vi "SetOpenDataEvents.vi"(7 "data group":string, 8 "error in (no error)":errorcluster, 9 "data event configs":T1[](array[typedef]), 10 "data events":T8[](array[typedef]), 11 "config":T7) -> (0 "error out":errorcluster, 3 "config out":T7)   [LabVIEW 2017, in "CmsDataEventCreator.lvlib"]
uses:
  <vilib>/addons/InsightCM/Devices/Shared/Cms/CmsDataEventCreator/CmsDataEventCreator.lvlib
  <vilib>/addons/InsightCM/Devices/Shared/Common/DataEvent/controls/Event.ctl
  <vilib>/addons/InsightCM/MessageBus/Base/controls/DataEvent.ctl
  <vilib>/addons/InsightCM/MessageBus/Base/controls/KeyValuePair.ctl
  <vilib>/addons/InsightCM/Devices/Shared/Common/DataEvent/controls/DataSet.ctl
  <vilib>/addons/InsightCM/MessageBus/Base/controls/DataSetMetadata.ctl
  <vilib>/addons/InsightCM/MessageBus/Base/controls/TrendPoint.ctl
  <vilib>/addons/InsightCM/MessageBus/Base/controls/TrendAlarmUpdate.ctl
  <vilib>/addons/InsightCM/MessageBus/Base/controls/TrendAlarmTransition.ctl
  <vilib>/addons/InsightCM/Devices/Shared/Cms/CmsDataEventCreator/controls/config.ctl
  <vilib>/addons/InsightCM/Devices/Shared/Cms/CmsDataEventCreator/controls/DataEventConfig.ctl
  <vilib>/addons/InsightCM/Devices/Shared/Cms/CmsDataEventCreator/controls/AcqParams.ctl
  <vilib>/addons/InsightCM/Devices/Shared/Common/DataAccumulator/controls/AccumulationSettings.ctl
  <vilib>/addons/InsightCM/Devices/Shared/Common/DataAccumulator/controls/accumulationType.ctl
  <vilib>/addons/InsightCM/Devices/Shared/Common/DVRBuffer/controls/BufferLocation.ctl
  <vilib>/addons/PointValueMap/controls/PointMap.ctl
  <vilib>/addons/InsightCM/Devices/Shared/Common/DataEvent/DataEvent.lvlib
  <vilib>/addons/InsightCM/Devices/Shared/Common/DataAccumulator/DataAccumulator.lvlib
  <vilib>/addons/InsightCM/Devices/Shared/Common/DVRBuffer/DVRBuffer.lvlib
  <vilib>/addons/PointValueMap/PointValueMap.lvlib
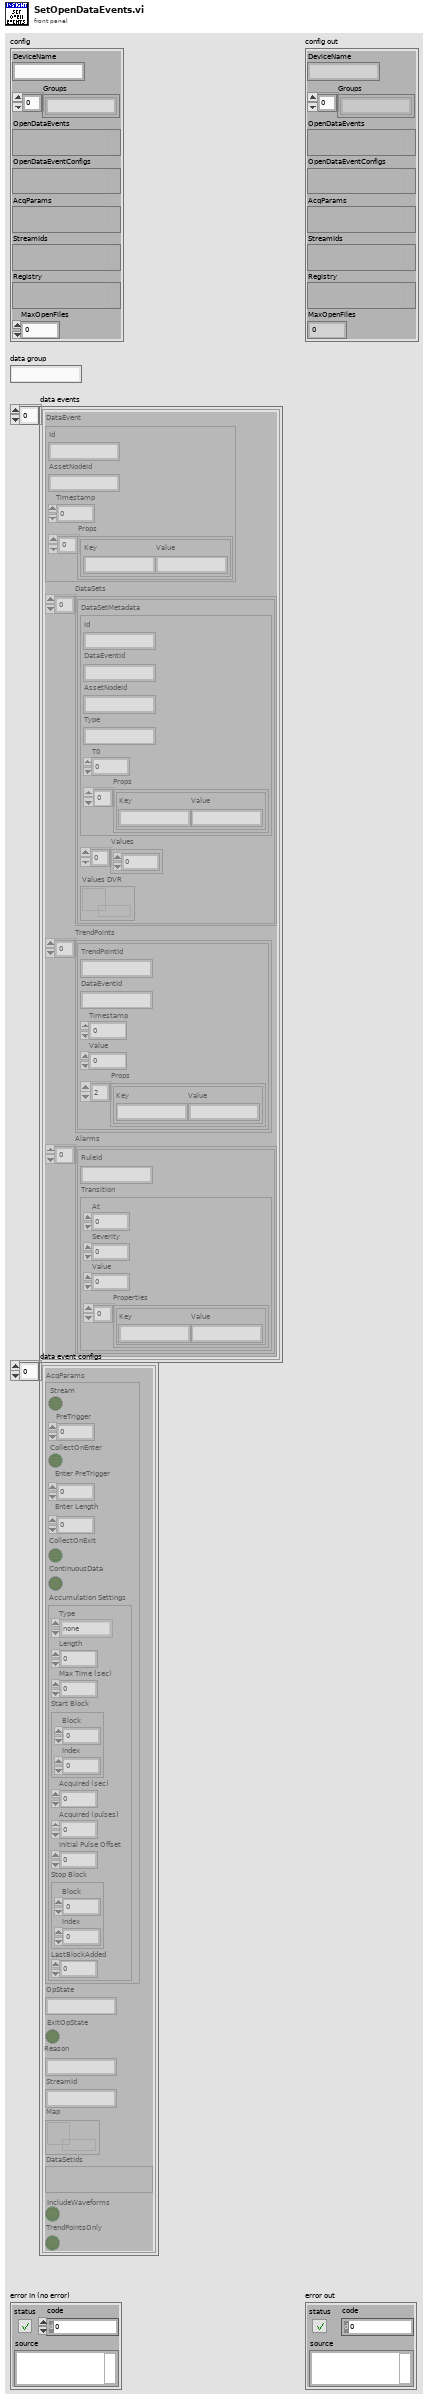
[diagram p1: front panel]
types:
  T1 = typedef "CmsDataEventCreator.lvlib/DataEventConfig.ctl" = cluster{"AcqParams":T2, "OpState":string, "ExitOpState":bool, "Reason":string, "StreamId":string, "Map":T6, "DataSetIds":variant, "IncludeWaveforms":bool, "TrendPointsOnly":bool}
  T2 = typedef "CmsDataEventCreator.lvlib/AcqParams.ctl" = cluster{"Stream":bool, "PreTrigger":i32, "CollectOnEnter":bool, "Enter PreTrigger":i32, "Enter Length":dbl, "CollectOnExit":bool, "ContinuousData":bool, "Accumulation Settings":T3}
  T3 = typedef "DataAccumulator.lvlib/AccumulationSettings.ctl" = cluster{"Type":T4, "Length":dbl, "Max Time (sec)":dbl, "Start Block":T5, "Acquired (sec)":dbl, "Acquired (pulses)":i32, "Initial Pulse Offset":dbl, "Stop Block":T5, "LastBlockAdded":u32}
  T4 = typedef "DataAccumulator.lvlib/accumulationType.ctl" = enum16{"none", "seconds", "revolutions"}
  T5 = typedef "DVRBuffer.lvlib/BufferLocation.ctl" = cluster{"Block":u32, "Index":i32}
  T6 = typedef "PointValueMap.lvlib/PointMap.ctl" = refnum<data-value>
  T7 = typedef "CmsDataEventCreator.lvlib/config.ctl" = cluster{"DeviceName":string, "Groups":string[], "OpenDataEvents":variant, "OpenDataEventConfigs":variant, "AcqParams":variant, "StreamIds":variant, "Registry":variant, "MaxOpenFiles":i32}
  T8 = typedef "DataEvent.lvlib/Event.ctl" = cluster{"DataEvent":T9, "DataSets":T11[], "TrendPoints":T13[], "Alarms":T14[]}
  T9 = typedef "DataEvent.ctl" = cluster{"Id":string, "AssetNodeId":string, "Timestamp":i64, "Props":T10[]}
  T10 = typedef "KeyValuePair.ctl" = cluster{"Key":string, "Value":string}
  T11 = typedef "DataEvent.lvlib/DataSet.ctl" = cluster{"DataSetMetadata":T12, "Values":sgl[], "Values DVR":refnum<data-value>}
  T12 = typedef "DataSetMetadata.ctl" = cluster{"Id":string, "DataEventId":string, "AssetNodeId":string, "Type":string, "T0":i64, "Props":T10[]}
  T13 = typedef "TrendPoint.ctl" = cluster{"TrendPointId":string, "DataEventId":string, "Timestamp":i64, "Value":dbl, "Props":T10[]}
  T14 = typedef "TrendAlarmUpdate.ctl" = cluster{"RuleId":string, "Transition":T15}
  T15 = typedef "TrendAlarmTransition.ctl" = cluster{"At":i64, "Severity":i32, "Value":dbl, "Properties":T10[]}
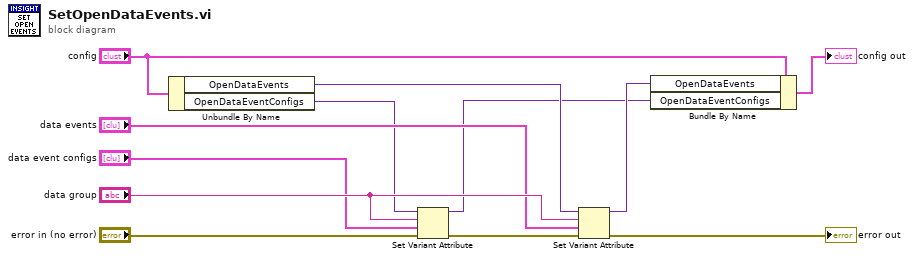
[diagram p0: block diagram]
diagram:
  n1 = Unbundle By Name("config") -> ("OpenDataEvents"=w6:variant, "OpenDataEventConfigs"=w5:variant)
  n2 = Set Variant Attribute(Variant=w5, name="data group", value="data event configs", error in="error in (no error)") -> (Variant out=w2:variant, error out=→"error out":errorcluster)  [unwired: 1 out]
  n3 = Set Variant Attribute(Variant=w6, name="data group", value="data events") -> (Variant out=w3:variant)  [unwired: 1 in, 2 out]
  n4 = Bundle By Name(cluster="config", "OpenDataEvents"=w3, "OpenDataEventConfigs"=w2) -> (→"config out":T7)
